vi "DSF.Engine.BuilderManager.Builder FIFO.Destroy.vi"(8 "error in (no error)":errorcluster, 11 "Builder Manager in":refnum<class "DSF.Engine.BuilderManager.lvclass">) -> (0 "error out":errorcluster, 3 "Builder Manager out":refnum<class "DSF.Engine.BuilderManager.lvclass">)   [LabVIEW 2017, in "DSF.Engine.lvlib" / "DSF.Engine.BuilderManager.lvclass"]
uses:
  DSF.Engine.BuilderManager.lvclass
  DSF.Engine.BuilderManager.lvclass/DSF.Engine.BuilderManager.ctl
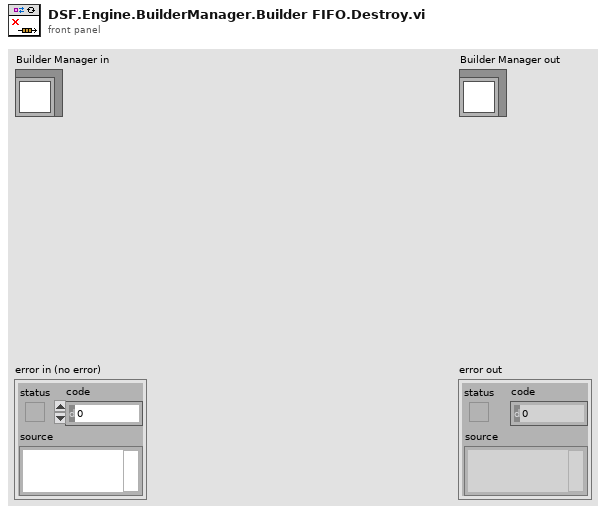
[diagram p1: front panel]
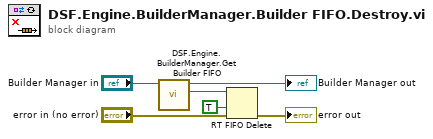
[diagram p0: block diagram]
diagram:
  n1 = call "DSF.Engine.BuilderManager.Get Builder FIFO.vi"("Builder Manager in"="Builder Manager in") -> ("Builder FIFO"=w5:refnum<k33>, "Builder Manager out"=→"Builder Manager out":refnum<class "DSF.Engine.BuilderManager.lvclass">)  [unwired: 9 in]
  n2 = RT FIFO Delete(0:w5, 2:TRUE ("force destroy? (F)"), 3:"error in (no error)") -> (11:→"error out":errorcluster)
